vi "nmea.vi"(8 "ecef ref":dbl[](array[numeric]) format="%#_19f", 11 "NMEA":string) -> (0 "output":dbl[](array[numeric]) format="%#_19f", 3 "type":u32)   [LabVIEW 2015]
uses:
  <vilib>/Analysis/Matrix/Numeric/Conversions/Array To Matrix - RA.vi
  <vilib>/Analysis/Matrix/Numeric/Conversions/Array To Matrix - RA2.vi
  <vilib>/Analysis/Matrix/Numeric/Multiply/Multiply - RM,RM.vi
  <vilib>/Analysis/Matrix/Numeric/Conversions/Matrix To Array - RM.vi
  <vilib>/Analysis/Matrix/NI_Matrix.lvlib
panel:
  out "trk gnd":dbl
  out "speed":dbl
  out "sol stat":i16
  out "ms rmc":dbl format="%#_6f"
  out "lat rmc":dbl format="%#_12f"
  out "lon rmc":dbl format="%#_12f"
  out "ecef":dbl[](array[numeric]) format="%#_19f"
  out "DCM(ecef2lcc)":dbl[][](array[numeric])
  out "diff_age":i32
  out "hgt":i32
  out "dev":dbl
  out "#SV":i32
  out "pos type":i32
  out "lon":dbl format="%#_12f"
  out "lat":dbl format="%#_12f"
  out "ms":dbl format="%#_6f"
  out "chksum":bool
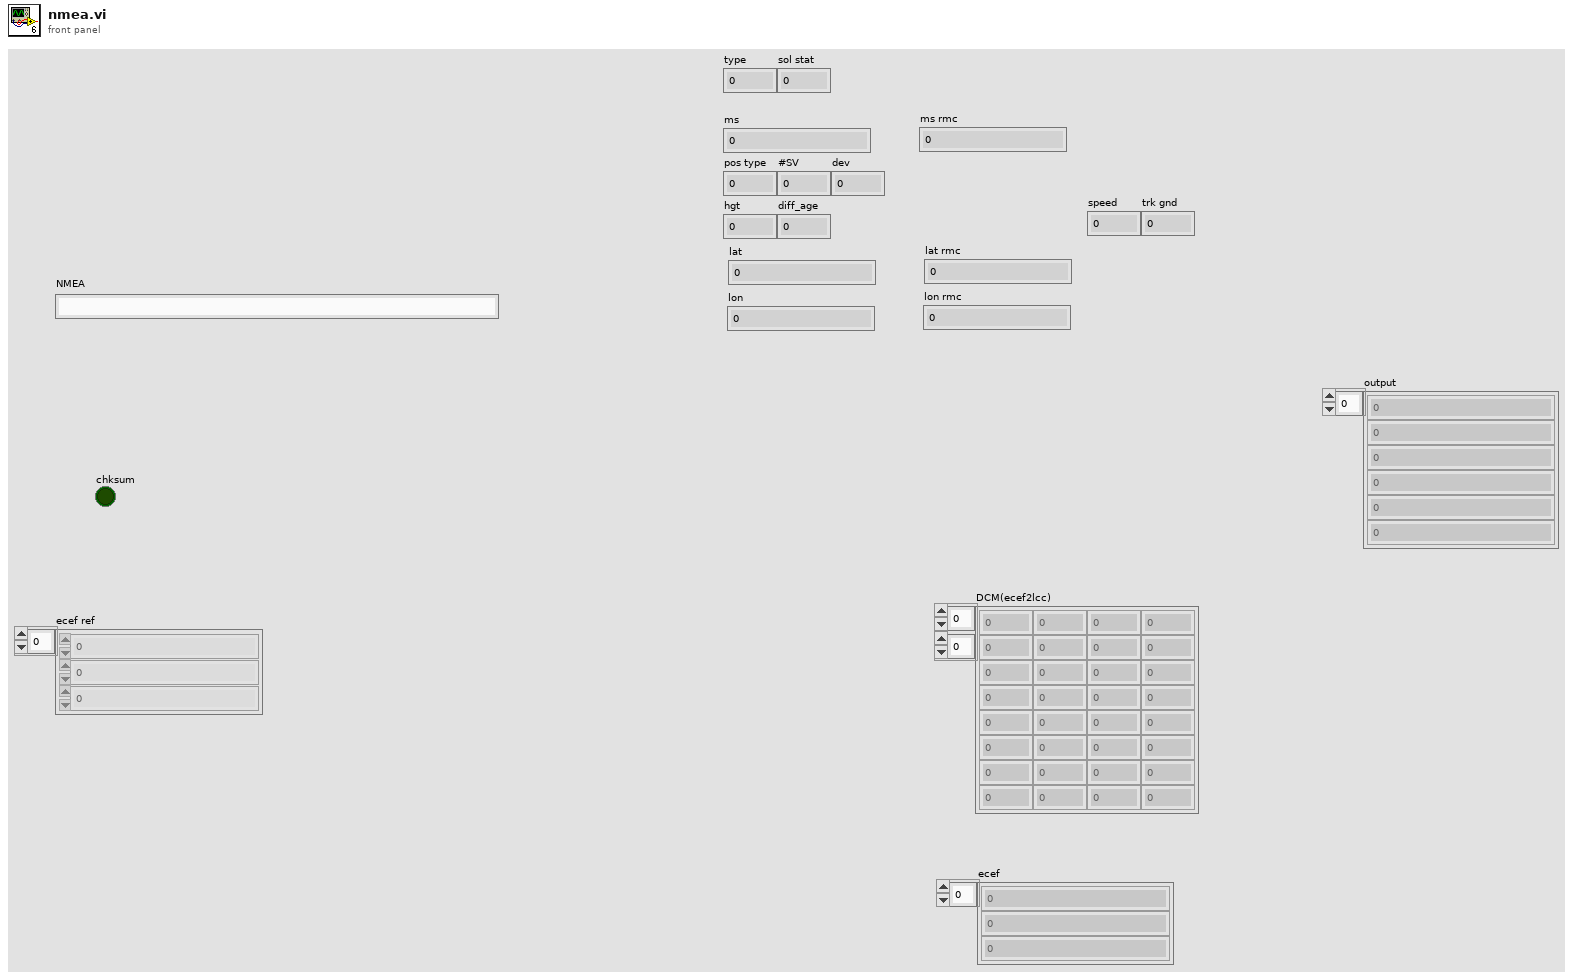
[diagram p1: front panel]
types:
  T1 = typedef "NI_Matrix.lvlib/RealMatrix.ctl" = dbl[][]
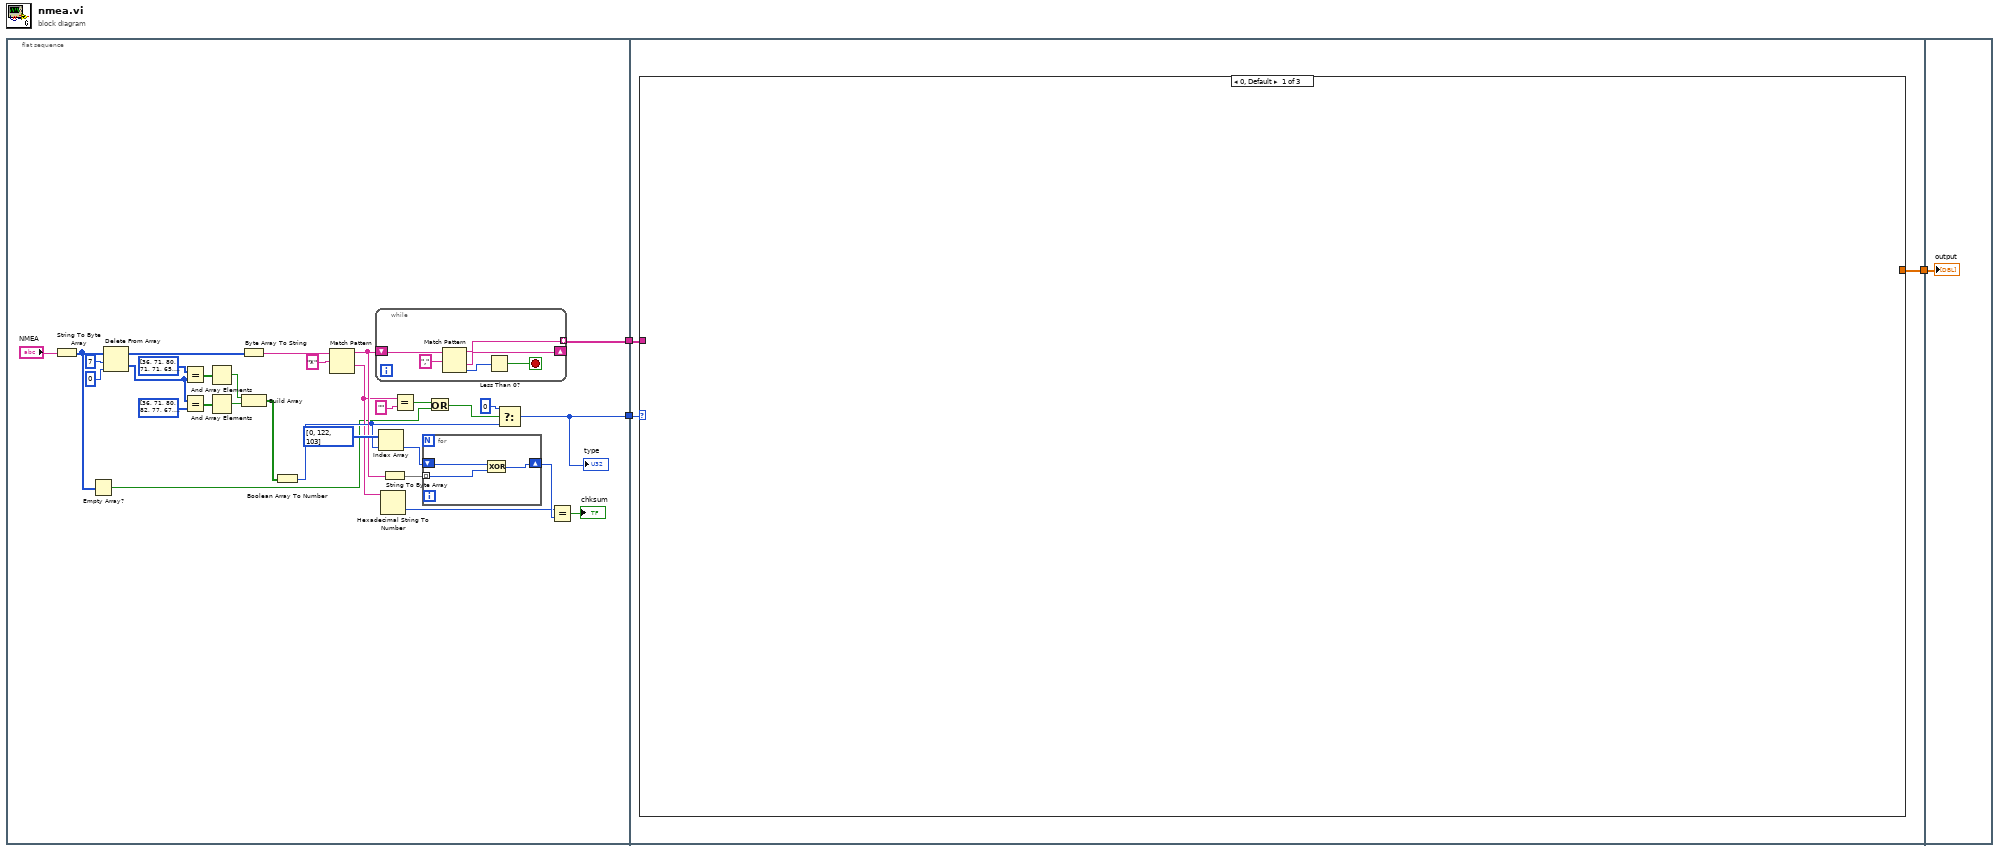
[diagram p0: block diagram]
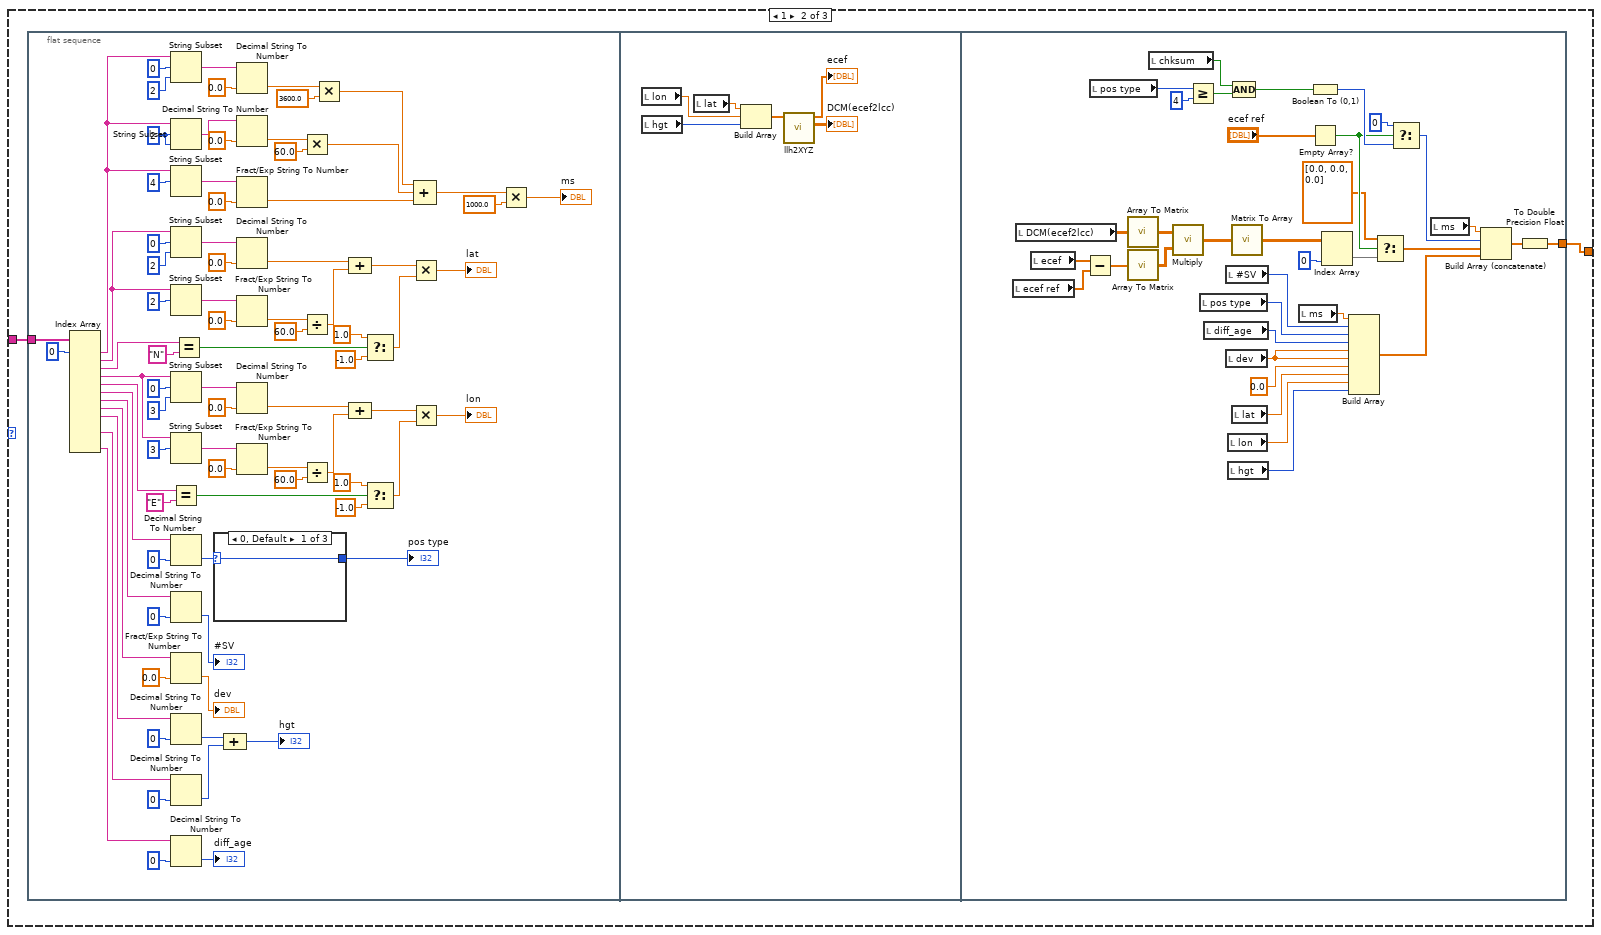
[diagram p2: hidden frame]
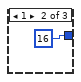
[diagram p3: hidden frame]
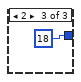
[diagram p4: hidden frame]
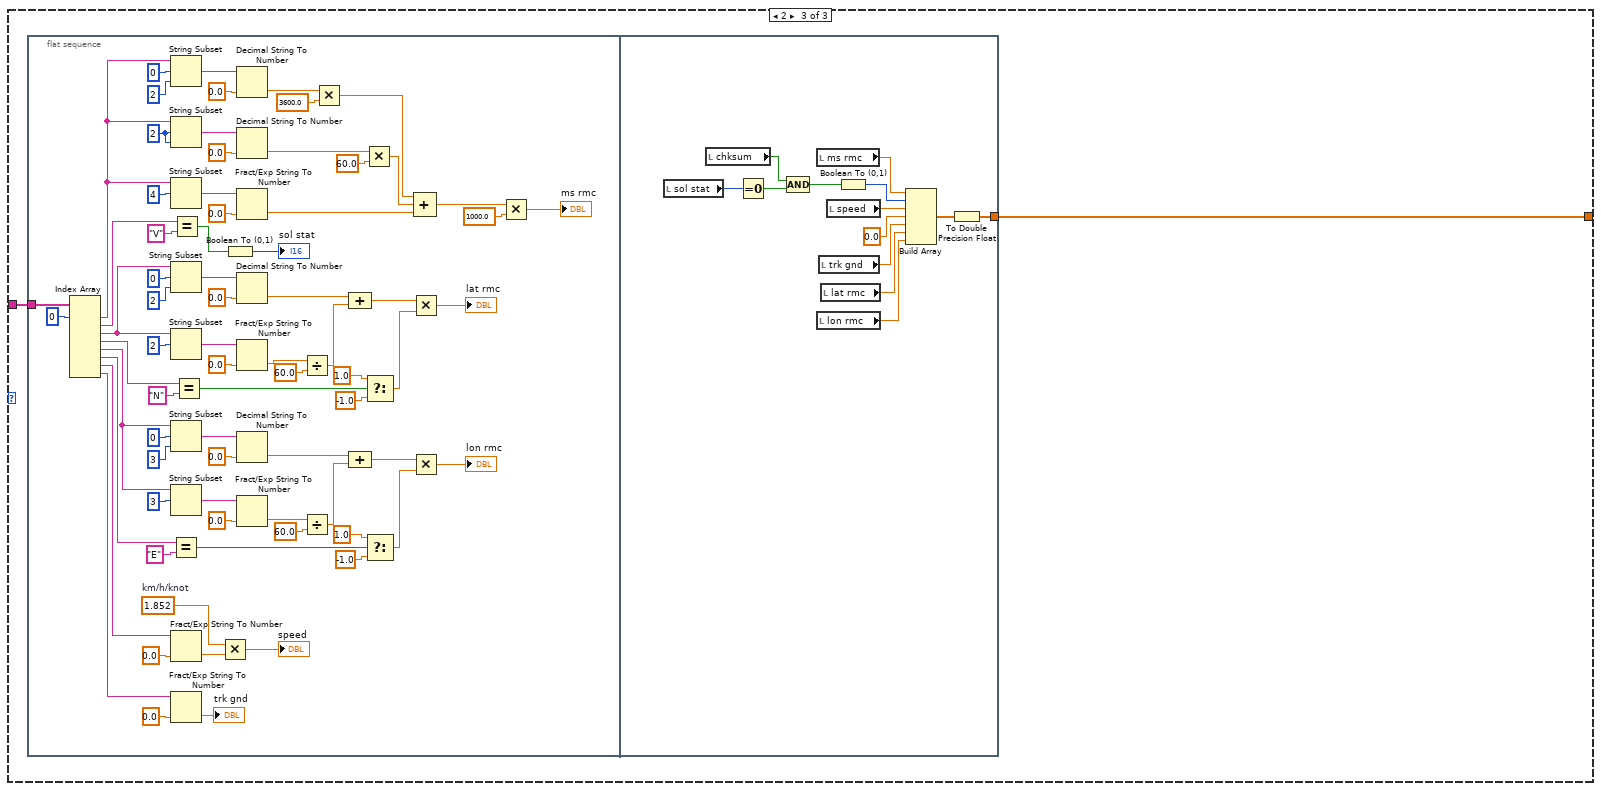
[diagram p5: hidden frame]
diagram:
  n1 = flat-sequence {
    tunnel: [w13] -> w3
    tunnel: [w4] -> w2
    tunnel: w3 -> [w46]
    tunnel: w2 -> [w45]
    tunnel: [w44] -> w1
    tunnel: w1 -> [w266]
    frame #0 {
      n2 = String To Byte Array(string="NMEA") -> (unsigned byte array=w12:u8[])
      n3 = Empty Array?(array=w12) -> (empty?=w6:bool)
      n4 = Delete From Array(array=w12, length=7, index=0) -> (deleted portion=w14:u8[], array with subset deleted=w32:u8[])
      n5 = Equal?(x=u8[] [36, 71, 80, 71, 71, 65, 44] ("gpgga"), y=w14) -> (x = y?=w31:bool[])
      n6 = Equal?(x=w14, y=u8[] [36, 71, 80, 82, 77, 67, 44] ("gprmc")) -> (x = y?=w26:bool[])
      n7 = And Array Elements(Boolean array=w31) -> (logical AND=w30:bool)
      n8 = And Array Elements(Boolean array=w26) -> (logical AND=w16:bool)
      n9 = Byte Array To String(unsigned byte array=w32) -> (string=w28:string)
      n10 = Build Array(w30, w16) -> (w29:bool[])
      n11 = Boolean Array To Number(Boolean array=w29) -> (number=w11:u32)
      n12 = Match Pattern(string=w28, regular expression="*") -> (before substring=w22:string, after substring=w9:string)  [unwired: 1 in, 2 out]
      n13 = while {
        shift-right: [w42] -> _
        shift-left: w22 -> [w43]
        tunnel: [w40] -> w13 mode=indexing
        stop <- w38 stop-if-true
        n14 = Match Pattern(string=w43, regular expression=",") -> (before substring=w40:string, after substring=w42:string, offset past match=w39:i32)  [unwired: 1 in, 1 out]
        n15 = Less Than 0?(x=w39) -> (x < 0?=w38:bool)
      }
      n16 = Index Array(array=u8[] [0, 122, 103], index=w11) -> (element=w19:u8)
      n17 = Hexadecimal String To Number(string=w9) -> (number=w17:u32)  [unwired: 2 in, 1 out]
      n18 = String To Byte Array(string=w22) -> (unsigned byte array=w21:u8[])
      n19 = Equal?(x=w9, y="") -> (x = y?=w7:bool)
      n20 = for {
        tunnel: w21 -> [w36] mode=indexing
        shift-right: [w35] -> w18
        shift-left: w19 -> [w37]
        n21 = Exclusive Or(1:w36, 2:w37) -> (0:w35:u8)
      }
      n22 = Or(x=w7, y=w6) -> (x .or. y?=w5:bool)
      n23 = Select(t=u32 0, s=w5, f=w11) -> (s? t:f=w4:u32)
      "type" <- w4
      n24 = Equal?(x=w17, y=w18) -> (x = y?=→"chksum":bool)
    }
    frame #1 {
      n25 = case shown="0, Default" w45 {
        tunnel: w46 -> [_ w48 w177]
        tunnel: [_ w47 w176] -> w44
        frame 0, Default {
        }
        frame 1 {
          n26 = flat-sequence {
            tunnel: w48 -> [w131]
            tunnel: [w141] -> w47
            frame #0 {
              w127 = 2 ("length (rest)")
              n27 = Index Array(array=w131, index #1=0 ("index")) -> (element #1=w98:string, element #2=w97:string, element #3=w96:string, element #4=w70:string, element #5=w69:string, element #6=w68:string, element #7=w63:string, element #8=w60:string, element #9=w57:string, element #11=w55:string, element #13=w50:string)  [unwired: 12 in, 2 out]
              n28 = String Subset(string=w98, offset (0)=0, length (rest)=2 ("length (rest)")) -> (substring=w125:string)
              n29 = String Subset(string=w98, offset (0)=w127, length (rest)=w127) -> (substring=w119:string)
              n30 = String Subset(string=w98, offset (0)=4) -> (substring=w115:string)  [unwired: 1 in]
              n31 = String Subset(string=w97, offset (0)=0, length (rest)=2 ("length (rest)")) -> (substring=w106:string)
              n32 = String Subset(string=w97, offset (0)=2) -> (substring=w108:string)  [unwired: 1 in]
              n33 = String Subset(string=w70, offset (0)=0, length (rest)=3 ("length (rest)")) -> (substring=w74:string)
              n34 = String Subset(string=w70, offset (0)=3) -> (substring=w72:string)  [unwired: 1 in]
              n35 = Equal?(x=w69, y="E") -> (x = y?=w83:bool)
              n36 = Decimal String To Number(string=w68, default (0L)=0 ("default (0 I32)")) -> (number=w66:i32)  [unwired: 1 in, 1 out]
              n37 = Decimal String To Number(string=w63, default (0L)=0 ("default (0 I32)")) -> (number=→"#SV":i32)  [unwired: 1 in, 1 out]
              n38 = Fract/Exp String To Number(string=w60, default (0 dbl)=0.0 ("default (0 I32)")) -> (number=→"dev":dbl)  [unwired: 2 in, 1 out]
              n39 = Decimal String To Number(string=w57, default (0L)=0 ("default (0 I32)")) -> (number=w54:i32)  [unwired: 1 in, 1 out]
              n40 = Decimal String To Number(string=w55, default (0L)=0 ("default (0 I32)")) -> (number=w53:i32)  [unwired: 1 in, 1 out]
              n41 = Decimal String To Number(string=w50, default (0L)=0 ("default (0 I32)")) -> (number=→"diff_age":i32)  [unwired: 1 in, 1 out]
              n42 = Equal?(x=w96, y="N") -> (x = y?=w94:bool)
              n43 = case shown="0, Default" w66 {
                selector: w66 -> [w132 _ _]
                tunnel: [w132 16 18] -> w65
                frame 0, Default {
                }
                frame 1 {
                }
                frame 2 {
                }
              }
              "pos type" <- w65
              n44 = Compound Arithmetic op=ADD(w54, w53) -> (→"hgt":i32)
              n45 = Decimal String To Number(string=w125, default (0L)=0.0 ("default (0 I32)")) -> (number=w124:dbl)  [unwired: 1 in, 1 out]
              n46 = Decimal String To Number(string=w119, default (0L)=0.0 ("default (0 I32)")) -> (number=w120:dbl)  [unwired: 1 in, 1 out]
              n47 = Fract/Exp String To Number(string=w115, default (0 dbl)=0.0 ("default (0 I32)")) -> (number=w113:dbl)  [unwired: 2 in, 1 out]
              n48 = Decimal String To Number(string=w106, default (0L)=0.0 ("default (0 I32)")) -> (number=w102:dbl)  [unwired: 1 in, 1 out]
              n49 = Fract/Exp String To Number(string=w108, default (0 dbl)=0.0 ("default (0 I32)")) -> (number=w101:dbl)  [unwired: 2 in, 1 out]
              n50 = Decimal String To Number(string=w74, default (0L)=0.0 ("default (0 I32)")) -> (number=w78:dbl)  [unwired: 1 in, 1 out]
              n51 = Fract/Exp String To Number(string=w72, default (0 dbl)=0.0 ("default (0 I32)")) -> (number=w79:dbl)  [unwired: 2 in, 1 out]
              n52 = Multiply(x=w120, y=60.0) -> (x*y=w116:dbl)
              n53 = Divide(x=w101, y=60.0) -> (x/y=w99:dbl)
              n54 = Divide(x=w79, y=60.0) -> (x/y=w81:dbl)
              n55 = Multiply(x=w124, y=3600.0) -> (x*y=w117:dbl)
              n56 = Compound Arithmetic op=ADD(w102, w99) -> (w91:dbl)
              n57 = Compound Arithmetic op=ADD(w78, w81) -> (w86:dbl)
              n58 = Select(t=1.0, s=w94, f=-1.0) -> (s? t:f=w90:dbl)
              n59 = Select(t=1.0, s=w83, f=-1.0) -> (s? t:f=w87:dbl)
              n60 = Multiply(x=w91, y=w90) -> (x*y=→"lat":dbl)
              n61 = Multiply(x=w86, y=w87) -> (x*y=→"lon":dbl)
              n62 = Compound Arithmetic op=ADD(w117, w116, w113) -> (w112:dbl)
              n63 = Multiply(x=w112, y=1000.0) -> (x*y=→"ms":dbl)
            }
            frame #1 {
              n64 = local read "lon"() -> (w139:dbl)
              n65 = local read "hgt"() -> (w138:i32)
              n66 = local read "lat"() -> (w140:dbl)
              n67 = Build Array(w140, w139, w138) -> (w137:dbl[])
              n68 = call "llh2XYZ.vi"("llh"=w137) -> ("DCM(ecef2lcc)"=→"DCM(ecef2lcc)":dbl[][], "ecef"=→"ecef":dbl[])  [unwired: 7 in]
            }
            frame #2 {
              n69 = local read "ecef ref"() -> (w157:dbl[])
              n70 = local read "DCM(ecef2lcc)"() -> (w158:dbl[][])
              n71 = local read "ecef"() -> (w156:dbl[])
              n72 = Subtract(x=w156, y=w157) -> (x-y=w160:dbl[])
              n73 = local read "pos type"() -> (w151:i32)
              n74 = call-poly <vilib>:"Array To Matrix.vi"("Real 2D Array"=w158) -> ("Real Matrix"=w159:T1)
              n75 = call-poly <vilib>:"Array To Matrix.vi"("Real 1D Array"=w160) -> ("Real Matrix (Column Vector)"=w161:T1)
              n76 = local read "chksum"() -> (w150:bool)
              n77 = call-poly <vilib>:"Multiply.vi"("Real Matrix B"=w161, "Real Matrix A"=w159) -> ("A * B"=w162:T1)
              n78 = Greater Or Equal?(x=w151, y=u32 4) -> (x >= y?=w167:bool)
              n79 = local read "pos type"() -> (w148:i32)
              n80 = local read "diff_age"() -> (w147:i32)
              n81 = local read "#SV"() -> (w149:i32)
              n82 = local read "dev"() -> (w146:dbl)
              n83 = local read "lon"() -> (w143:dbl)
              n84 = local read "hgt"() -> (w142:i32)
              n85 = call-poly <vilib>:"Matrix To Array.vi"("Real Matrix"=w162) -> ("Real 2D Array"=w163:dbl[][])
              n86 = local read "lat"() -> (w144:dbl)
              n87 = Compound Arithmetic op=AND(w150, w167) -> (w168:bool)
              n88 = local read "ms"() -> (w152:dbl)
              n89 = Boolean To (0,1)(Boolean=w168) -> (0, 1=w173:i16)
              n90 = Empty Array?(array="ecef ref") -> (empty?=w172:bool)
              n91 = Index Array(array=w163, index (col)=0 ("disabled index (col)")) -> (element=w170:dbl[])  [unwired: 1 in]
              n92 = Build Array(w152, w149, w148, w147, w146, w146, 0.0 ("element"), w144, w143, w142) -> (w169:dbl[])
              n93 = Select(t=dbl[] [0.0, 0.0, 0.0] ("subarray"), s=w172, f=w170) -> (s? t:f=w171:dbl[])
              n94 = Select(t=i16 0, s=w172, f=w173) -> (s? t:f=w174:i16)
              n95 = local read "ms"() -> (w153:dbl)
              n96 = Build Array (concatenate)(w153, w174, w171, w169) -> (w165:dbl[])
              n97 = To Double Precision Float(number=w165) -> (double precision float=w141:dbl[])
            }
          }
        }
        frame 2 {
          n98 = flat-sequence {
            tunnel: w177 -> [w252]
            tunnel: [w255] -> w176
            frame #0 {
              w179 = 1.852  # km/h/knot
              w249 = 2 ("length (rest)")
              n99 = Index Array(array=w252, index #1=0 ("index")) -> (element #1=w191:string, element #2=w189:string, element #3=w220:string, element #4=w219:string, element #5=w193:string, element #6=w192:string, element #7=w185:string, element #8=w181:string)  [unwired: 7 in]
              n100 = String Subset(string=w191, offset (0)=0, length (rest)=2 ("length (rest)")) -> (substring=w247:string)
              n101 = String Subset(string=w191, offset (0)=w249, length (rest)=w249) -> (substring=w241:string)
              n102 = String Subset(string=w191, offset (0)=4) -> (substring=w237:string)  [unwired: 1 in]
              n103 = String Subset(string=w220, offset (0)=0, length (rest)=2 ("length (rest)")) -> (substring=w228:string)
              n104 = String Subset(string=w220, offset (0)=2) -> (substring=w230:string)  [unwired: 1 in]
              n105 = String Subset(string=w193, offset (0)=0, length (rest)=3 ("length (rest)")) -> (substring=w197:string)
              n106 = String Subset(string=w193, offset (0)=3) -> (substring=w195:string)  [unwired: 1 in]
              n107 = Equal?(x=w192, y="E") -> (x = y?=w206:bool)
              n108 = Fract/Exp String To Number(string=w185, default (0 dbl)=0.0 ("default (0 I32)")) -> (number=w178:dbl)  [unwired: 2 in, 1 out]
              n109 = Fract/Exp String To Number(string=w181, default (0 dbl)=0.0 ("default (0 I32)")) -> (number=→"trk gnd":dbl)  [unwired: 2 in, 1 out]
              n110 = Equal?(x=w189, y="V") -> (x = y?=w187:bool)
              n111 = Equal?(x=w219, y="N") -> (x = y?=w217:bool)
              n112 = Multiply(x=w179, y=w178) -> (x*y=→"speed":dbl)
              n113 = Boolean To (0,1)(Boolean=w187) -> (0, 1=→"sol stat":i16)
              n114 = Decimal String To Number(string=w247, default (0L)=0.0 ("default (0 I32)")) -> (number=w246:dbl)  [unwired: 1 in, 1 out]
              n115 = Decimal String To Number(string=w241, default (0L)=0.0 ("default (0 I32)")) -> (number=w242:dbl)  [unwired: 1 in, 1 out]
              n116 = Fract/Exp String To Number(string=w237, default (0 dbl)=0.0 ("default (0 I32)")) -> (number=w235:dbl)  [unwired: 2 in, 1 out]
              n117 = Decimal String To Number(string=w228, default (0L)=0.0 ("default (0 I32)")) -> (number=w224:dbl)  [unwired: 1 in, 1 out]
              n118 = Fract/Exp String To Number(string=w230, default (0 dbl)=0.0 ("default (0 I32)")) -> (number=w223:dbl)  [unwired: 2 in, 1 out]
              n119 = Decimal String To Number(string=w197, default (0L)=0.0 ("default (0 I32)")) -> (number=w201:dbl)  [unwired: 1 in, 1 out]
              n120 = Fract/Exp String To Number(string=w195, default (0 dbl)=0.0 ("default (0 I32)")) -> (number=w202:dbl)  [unwired: 2 in, 1 out]
              n121 = Divide(x=w223, y=60.0) -> (x/y=w221:dbl)
              n122 = Divide(x=w202, y=60.0) -> (x/y=w204:dbl)
              n123 = Multiply(x=w246, y=3600.0) -> (x*y=w239:dbl)
              n124 = Compound Arithmetic op=ADD(w224, w221) -> (w214:dbl)
              n125 = Compound Arithmetic op=ADD(w201, w204) -> (w209:dbl)
              n126 = Multiply(x=w242, y=60.0) -> (x*y=w238:dbl)
              n127 = Select(t=1.0, s=w217, f=-1.0) -> (s? t:f=w213:dbl)
              n128 = Select(t=1.0, s=w206, f=-1.0) -> (s? t:f=w210:dbl)
              n129 = Multiply(x=w214, y=w213) -> (x*y=→"lat rmc":dbl)
              n130 = Multiply(x=w209, y=w210) -> (x*y=→"lon rmc":dbl)
              n131 = Compound Arithmetic op=ADD(w239, w238, w235) -> (w234:dbl)
              n132 = Multiply(x=w234, y=1000.0) -> (x*y=→"ms rmc":dbl)
            }
            frame #1 {
              n133 = local read "sol stat"() -> (w259:i16)
              n134 = local read "chksum"() -> (w262:bool)
              n135 = Equal To 0?(x=w259) -> (x = 0?=w263:bool)
              n136 = Compound Arithmetic op=AND(w262, w263) -> (w264:bool)
              n137 = local read "ms rmc"() -> (w260:dbl)
              n138 = local read "lon rmc"() -> (w253:dbl)
              n139 = local read "trk gnd"() -> (w256:dbl)
              n140 = local read "lat rmc"() -> (w254:dbl)
              n141 = local read "speed"() -> (w258:dbl)
              n142 = Boolean To (0,1)(Boolean=w264) -> (0, 1=w265:i16)
              n143 = Build Array(w260, w265, w258, 0.0 ("element"), w256, w254, w253) -> (w261:dbl[])
              n144 = To Double Precision Float(number=w261) -> (double precision float=w255:dbl[])
            }
          }
        }
      }
    }
    frame #2 {
      "output" <- w266
    }
  }
